vi "get initial information.vi"(8 "error in (no error)":errorcluster, 10 "channel":u16, 11 "CCDCamera in":refnum<class "Ixon_Ultra.lvclass">) -> (0 "error out":errorcluster, 3 "CCDCamera out":refnum<class "Ixon_Ultra.lvclass">)   [LabVIEW 2018, in "Ixon_Ultra.lvclass"]
uses:
  Ixon_Ultra.lvclass
  C:/Users/Denis/Desktop/S4ACS/S4ACS/Sim_CCD/Sim_CCD.lvclass
  Sim_CCD/Sim_CCD.lvclass
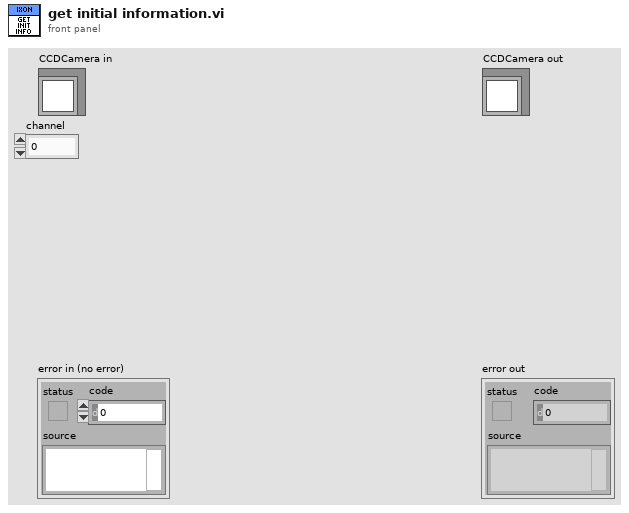
[diagram p1: front panel]
types:
  T1 = cluster{"FRAMES_DONE":u16, "CCD_STATUS":string, "CURRENT_TEMPERATURE":i16, "TEMPERATURE_STATUS":string, "FRAME_EXPOSURE_TIME":dbl, "SERIAL_NUMBER":u16, "ACQUIRING":bool, "POWER":bool, "ACS MODE":bool}
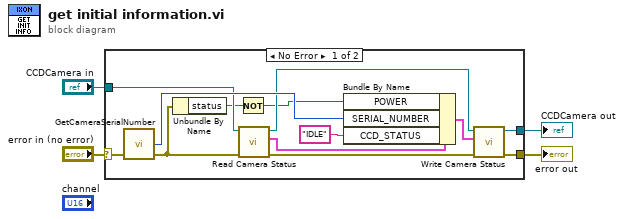
[diagram p0: block diagram]
diagram:
  n1 = case shown="No Error" "error in (no error)" {
    selector: "error in (no error)" -> [w10 w19]
    tunnel: "CCDCamera in" -> [w9 w18]
    tunnel: [w8 w18] -> w2
    tunnel: [w7 w19] -> w1
    frame No Error {
      n2 = call <userlib>:"GetCameraSerialNumber.vi"("error in (no error)"=w10) -> ("error out"=w11:errorcluster, "number"=w16:i32)  [unwired: 2 in, 1 out]
      n3 = Unbundle By Name(w11) -> ("status"=w6:bool)
      n4 = Not(x=w6) -> (.not. x?=w5:bool)
      n5 = call "Read Camera Status.vi"("error in (no error)"=w11, "CCDCamera in"=w9) -> ("error out"=w15:errorcluster, "camera status"=w13:T1, "CCDCamera out"=w14:refnum<class "Ixon_Ultra.lvclass">)  [unwired: 7 in]
      n6 = Bundle By Name(cluster=w13, "POWER"=w5, "SERIAL_NUMBER"=w16, "CCD_STATUS"="IDLE" ("Camera Status.STATUS")) -> (w12:T1)
      n7 = call "Write Camera Status.vi"("error in (no error)"=w15, "camera status"=w12, "CCDCamera in"=w14) -> ("error out"=w7:errorcluster, "CCDCamera out"=w8:refnum<class "Ixon_Ultra.lvclass">)  [unwired: 7 in]
    }
    frame Error {
    }
  }
  "error out" <- w1
  "CCDCamera out" <- w2
